vi "OpenBinData.vi"() -> ()   [LabVIEW 2013]
panel:
  out "data":dbl[](array[numeric])
  out "appended path":path
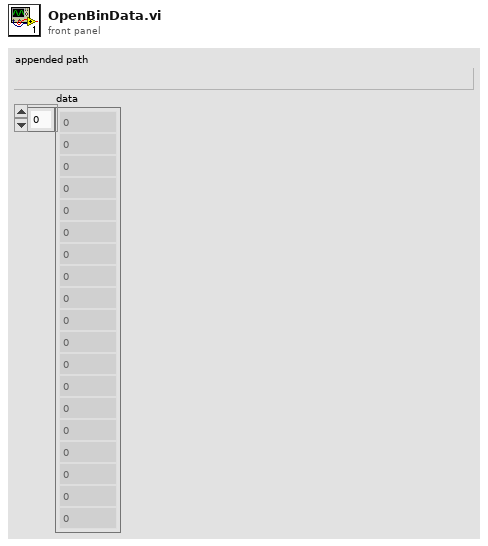
[diagram p1: front panel]
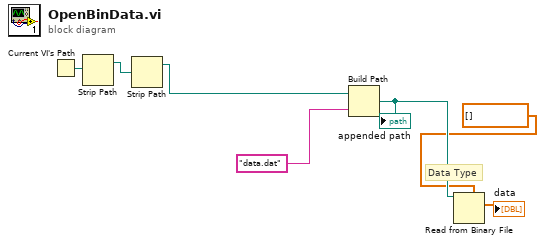
[diagram p0: block diagram]
diagram:
  # "Data Type"
  n1 = Current VI's Path() -> (path=w5:path)
  n2 = Strip Path(path=w5) -> (stripped path=w4:path)  [unwired: 1 out]
  n3 = Strip Path(path=w4) -> (stripped path=w3:path)  [unwired: 1 out]
  n4 = Build Path(base path=w3, name or relative path="data.dat") -> (appended path=w6:path)
  "appended path" <- w6
  n5 = Read from Binary File(5:dbl[] [], 11:w6) -> (2:→"data":dbl[])  [unwired: 4 in, 3 out]
